vi "Select_Alternative_channel.vi"(4 "Filetype":string, 5 "Extra Channel Values":string[][](array[string]), 6 "All Tabulated Channels":string[](array[string]), 7 "while Reading:":path, 9 "Template Channel Name":string, 10 "Data string":string, 11 "Previous Channels used":string[](array[string])) -> (0 "Chosen Channel":string, 3 "Selected Index":i32)   [LabVIEW 2021]
uses:
  83d2ac24-8169-844b-9428-30d31295317a.vi
panel:
  in  "Search":string
  in  "Cancel Button":bool
  out "Channel Values":dbl[](graph)
  out "Channel Values":string[](array[string])
  out "Message":string
  in  "Boolean":bool
  in  "Select channel to be used":i32(listbox)
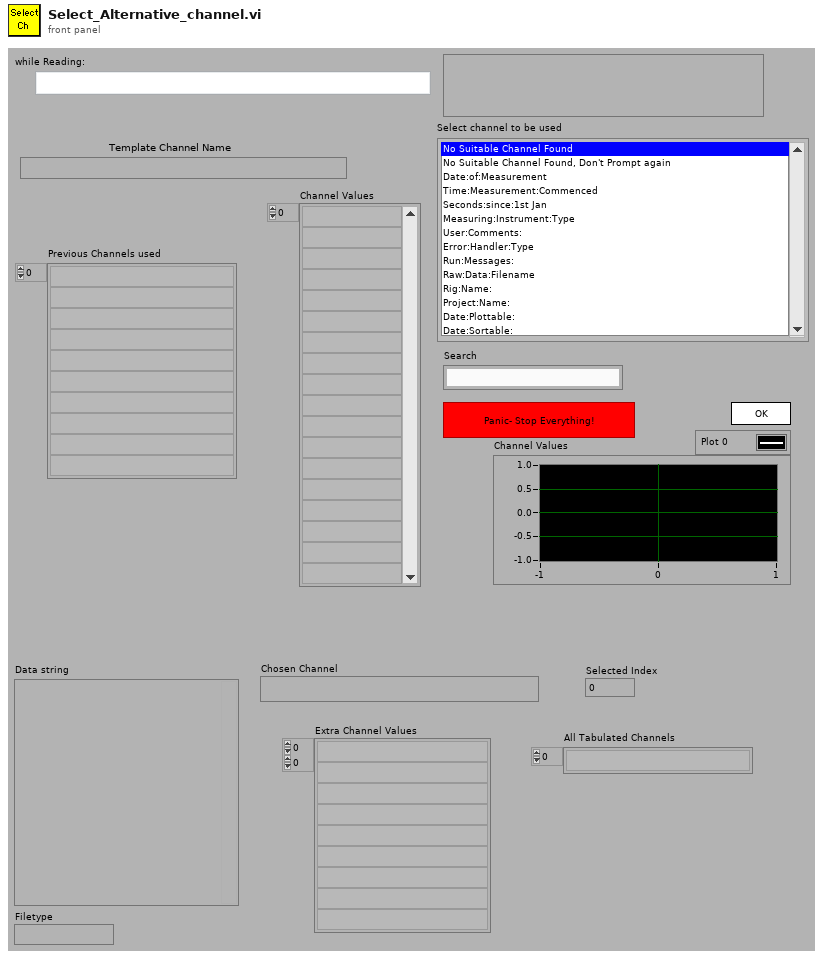
[diagram p1: front panel]
types:
  T1 = enum8{"Enabled", "Disabled", "Disabled and Grayed Out"}
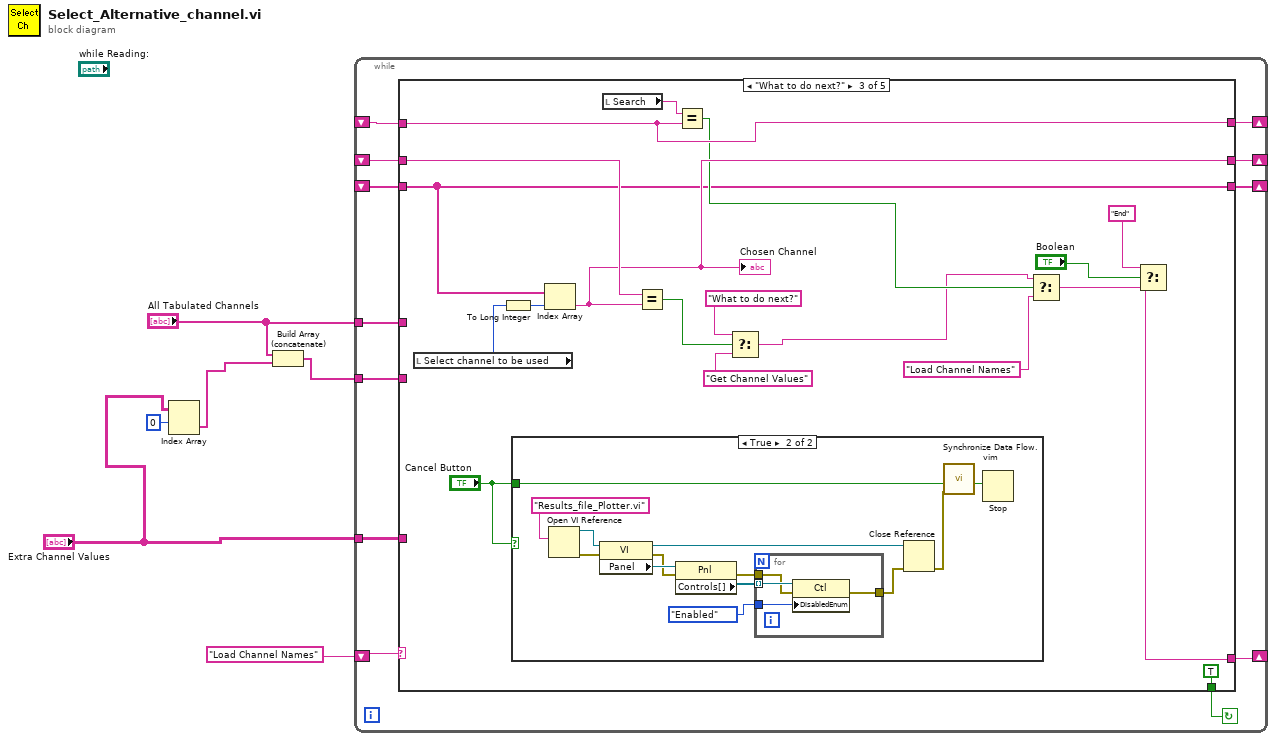
[diagram p0: block diagram]
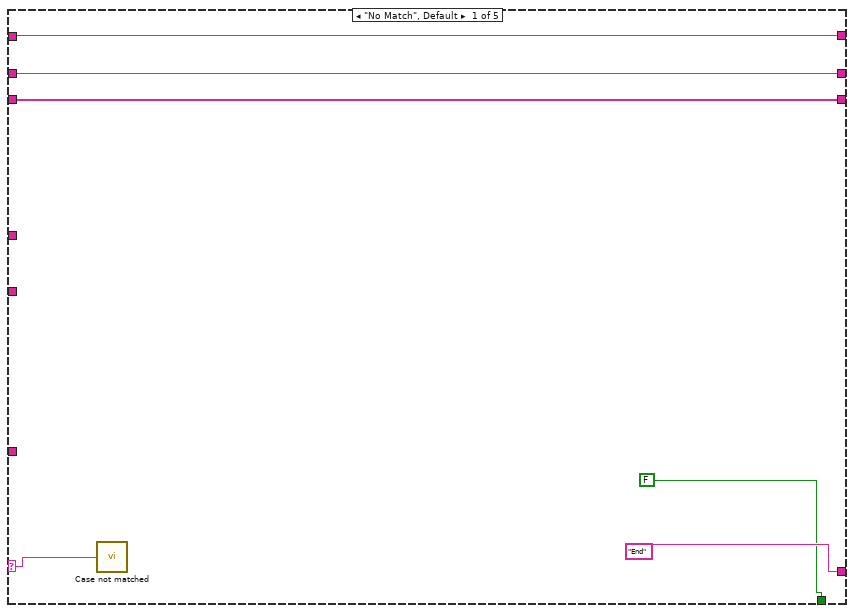
[diagram p2: hidden frame]
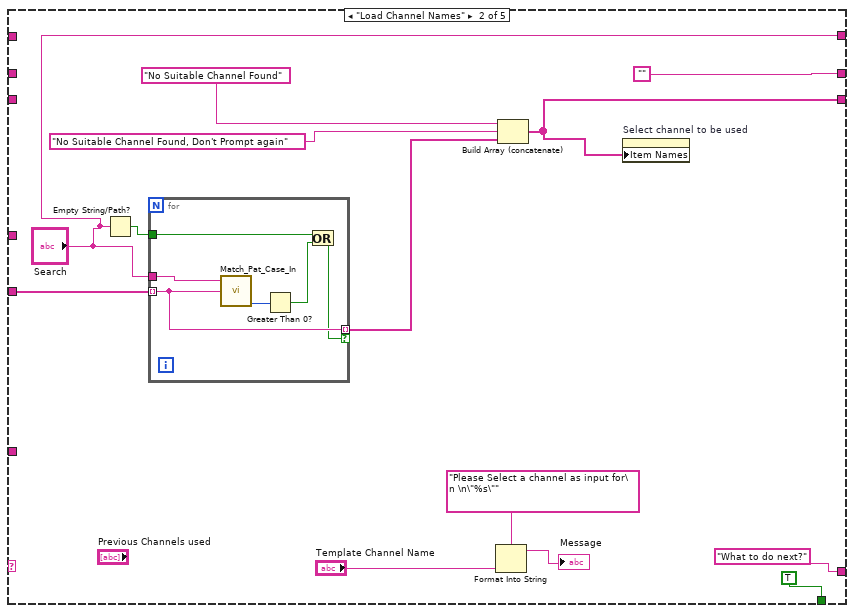
[diagram p3: hidden frame]
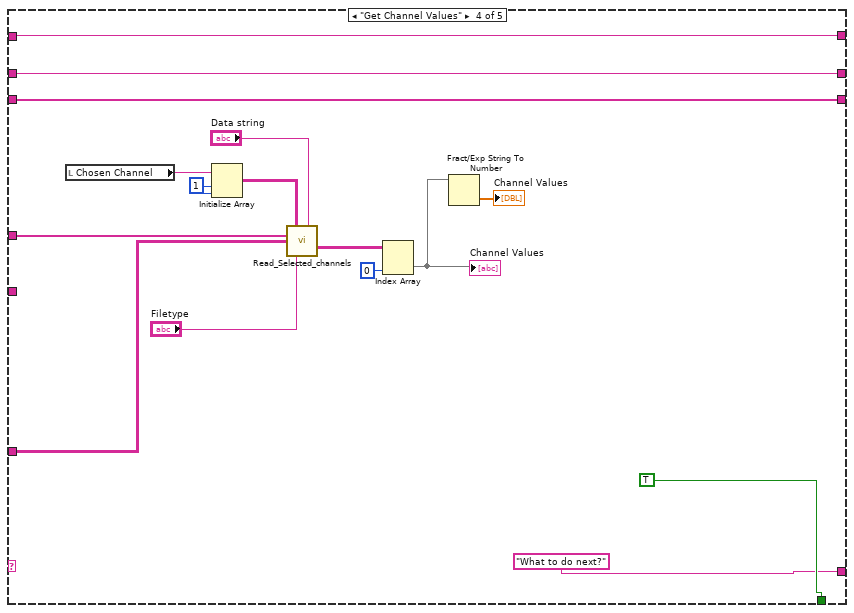
[diagram p5: hidden frame]
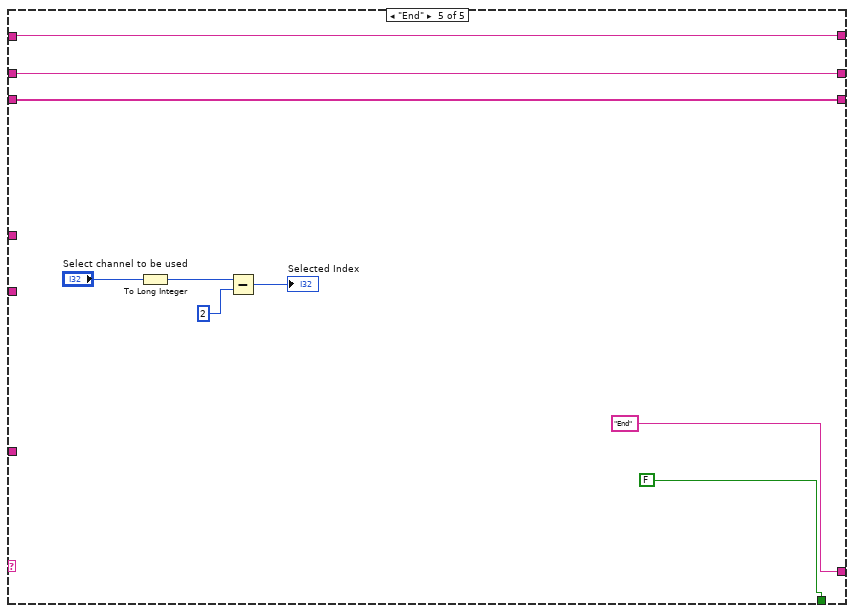
[diagram p6: hidden frame]
diagram:
  n1 = Index Array(array="Extra Channel Values", index (row)=0) -> (element=w1:string[])  [unwired: 1 in]
  n2 = Build Array (concatenate)("All Tabulated Channels", w1) -> (w5:string[])
  n3 = while {
    shift-left: "Load Channel Names" -> [w16]
    shift-right: [w17] -> _
    shift-right: [w14] -> _
    shift-left: _ -> [w15]
    shift-right: [w12] -> _
    shift-left: _ -> [w11]
    tunnel: w5 -> [w13]
    tunnel: "All Tabulated Channels" -> [w10]
    shift-right: [w9] -> _
    shift-left: _ -> [w8]
    tunnel: "Extra Channel Values" -> [w7]
    stop <- w18 continue-if-true
    n4 = case shown="\"What to do next?\"" w16 {
      selector: w16 -> [w19 _ _ _ _]
      tunnel: [FALSE TRUE TRUE TRUE FALSE] -> w18
      tunnel: ["End" "What to do next?" w59 "What to do next?" "End"] -> w17
      tunnel: w15 -> [w22 _ w56 w85 w99]
      tunnel: [w22 "" w55 w85 w99] -> w14
      tunnel: w13 -> [_ w29 _ _ _]
      tunnel: [w20 w26 w45 w82 w96] -> w12
      tunnel: w11 -> [w20 _ w45 w82 w96]
      tunnel: w10 -> [_ _ _ w83 _]
      tunnel: [w21 "Search" w50 w81 w97] -> w9
      tunnel: w8 -> [w21 _ w50 w81 w97]
      tunnel: w7 -> [_ _ _ w80 _]
      frame "No Match", Default {
        n5 = call "Case not matched.vi"("Case Name not Matched"=w19) -> ()
      }
      frame "Load Channel Names" {
        n6 = Empty String/Path?(string/path="Search") -> (empty?=w28:bool)
        n7 = for {
          tunnel: "Search" -> [w43]
          tunnel: w29 -> [w39] mode=indexing
          tunnel: w28 -> [w40]
          tunnel: [w39] -> w27 mode=indexing if=w38
          n8 = call "Match_Pat_Case_In.vi"("String to match"=w43, "String"=w39) -> ("offset past match"=w42:i32)  [unwired: 1 in, 3 out]
          n9 = Greater Than 0?(x=w42) -> (x > 0?=w41:bool)
          n10 = Or(x=w40, y=w41) -> (x .or. y?=w38:bool)
        }
        n11 = Format Into String(format string="Please Select a channel as input for\n \n\"%s\"" ("Format String"), "Template Channel Name") -> (resulting string=→"Message":string)  [unwired: 2 in, 1 out]
        n12 = Build Array (concatenate)("No Suitable Channel Found" ("Input Element"), "No Suitable Channel Found, Don't Prompt again" ("Input Element"), w27) -> (w26:string[])
        n13 = property on="Select channel to be used" class="LstBox (strict)"("Item Names"=w26) -> ()  [unwired: 2 in, 2 out]
      }
      frame "What to do next?" {
        n14 = local read "Select channel to be used"() -> (w62:i32)
        n15 = To Long Integer(number=w62) -> (32bit integer=w57:i32)
        n16 = case shown="True" "Cancel Button" {
          tunnel: "Cancel Button" -> [_ w75]
          frame False {
          }
          frame True {
            n17 = Open VI Reference(vi path="Results_file_Plotter.vi") -> (vi reference=w64:refnum<vi>, error out=w65:errorcluster)  [unwired: 5 in]
            n18 = property class="VI"(reference=w64, error in=w65) -> (reference out=w68:refnum<vi>, error out=w71:errorcluster, "Panel"=w74:refnum<vi>)
            n19 = property class="Pnl"(reference=w74, error in=w71) -> (error out=w70:errorcluster, "Controls[]"=w73:refnum<vi>[])  [unwired: 1 out]
            n20 = for {
              tunnel: w73 -> [w79] mode=indexing
              tunnel: T1."Enabled" ("Disabled") -> [w78]
              tunnel: w70 -> [w77]
              tunnel: [w76] -> w69
              n21 = property class="Ctl"(reference=w79, error in=w77, "DisabledEnum"=w78) -> (error out=w76:errorcluster)  [unwired: 1 out]
            }
            n22 = Close Reference(reference=w68, error in (no error)=w69) -> (error out=w66:errorcluster)
            n23 = call "Synchronize Data Flow.vim"("input 4"=w66, "input 3"=w75) -> ("output 3"=w67:bool)  [unwired: 2 in, 3 out]
            n24 = Stop(stop? (T)=w67) -> ()
          }
        }
        n25 = Index Array(array=w45, index=w57) -> (element=w55:string)
        "Chosen Channel" <- w55
        n26 = local read "Search"() -> (w51:string)
        n27 = Equal?(x=w56, y=w55) -> (x = y?=w52:bool)
        n28 = Equal?(x=w51, y=w50) -> (x = y?=w49:bool)
        n29 = Select(t="What to do next?", s=w52, f="Get Channel Values") -> (s? t:f=w48:string)
        n30 = Select(t=w48, s=w49, f="Load Channel Names") -> (s? t:f=w47:string)
        n31 = Select(t="End", s="Boolean", f=w47) -> (s? t:f=w59:string)
      }
      frame "Get Channel Values" {
        w93 = 1 ("dimension size")
        n32 = local read "Chosen Channel"() -> (w94:string)
        n33 = Initialize Array(w94, w93, w93) -> (w92:string[][])
        n34 = call "Read_Selected_channels.vi"("Valid Channel Options"=w92, "Data string"="Data string", "All Channels Present"=w83, "Extra Channels"=w80, "Filetype"="Filetype") -> ("Output Values"=w89:string[][])  [unwired: 4 in, 6 out]
        n35 = Index Array(array=w89, index (col)=0 ("index (row)")) -> (element=w88:string[])  [unwired: 1 in]
        "Channel Values" <- w88
        n36 = Fract/Exp String To Number(string=w88) -> (number=→"Channel Values":dbl[])  [unwired: 4 out]
      }
      frame "End" {
        n37 = To Long Integer(number="Select channel to be used") -> (32bit integer=w98:i32)
        n38 = Subtract(x=w98, y=2) -> (x-y=→"Selected Index":i32)
      }
    }
  }
